vi "Periodic Tasks.vi"(8 "error in":errorcluster) -> ()   [LabVIEW 2015]
doc: "This VI runs in parallel to other tasks. It can contain as many user-defined periodic loops as you need. These can carry out PID or other sorts of timed response."
uses:
  Common Code/Change Detect Int.vi
  Robot Global Data.vi
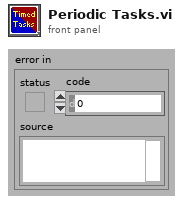
[diagram p1: front panel]
types:
  T1 = typedef "WPI_MotorControlDeviceRef.ctl" = cluster{"DeviceStatus":errorcluster, "Type":T2, "PWM":cluster{"PWM Channel":T3, "DeadBand":T4}, "CAN":cluster{"Device Number":u8, "Control Mode":T5, "Semaphore":T6, "Max Vout":dbl, "TalonSRX Control Mode":T7}, "Invert":bool}
  T2 = typedef "WPI_MotorControlType.ctl" = enum16{"PWM", "CAN", "CANTalonSRX"}
  T3 = typedef "FPGA_DIOPWMChannel.ctl" = enum8{"PWM 0", "PWM 1", "PWM 2", "PWM 3", "PWM 4", "PWM 5", "PWM 6", "PWM 7", "PWM 8", "PWM 9", "PWM MXP 0", "PWM MXP 1", "PWM MXP 2", "PWM MXP 3", "PWM MXP 4", "PWM MXP 5", "PWM MXP 6", "PWM MXP 7", "PWM MXP 8", "PWM MXP 9", "Invalid"}
  T4 = typedef "WPI_PWMDeadband.ctl" = cluster{"Name":string, "maxPositivePwm":i32, "minPositivePwm":i32, "centerPwm":i32, "maxNegativePwm":i32, "minNegativePwm":i32, "angularRange":u16}
  T5 = typedef "WPI_CANJaguar_ControlMode.ctl" = enum8{"Percent VBus", "Current", "Speed", "Position", "Voltage"}
  T6 = typedef "Semaphore RefNum" = refnum<k1>
  T7 = typedef "WPI_CANTalonSRX_APIControlMode.ctl" = enum8{"Percent VBus", "Speed", "Position", "Slave", "Unchanged / Invalid", "Voltage Compensation", "Current", "Motion Profile"}
  T8 = typedef "Dashboard Control Data.ctl" = cluster{"Shooter Presets":T9, "Encoder Control":T11, "Steer PID output":cluster{"output high":dbl, "output low":dbl}, " Steer PID gains":cluster{"proportional gain (Kc)":dbl, "integral time (Ti, min)":dbl, "derivative time (Td, min)":dbl}, "Drivetrain Settings":T12, "Vision Packet":T13, "Dashboard Drivetrain Command":T14, "Info/Command Cluster":T16, "Ball Vision Packet":T17, "Intake Presets":T19, "Intake Encoder Control":T21, "Climb Presets":T22, "Ultrasonic Limit":dbl, "Roll Limit":dbl, "Pitch Limit":dbl, "Goal Output Range":cluster{"output high":dbl, "output low":dbl}, "Enabled Systems":T23}
  T9 = typedef "Shooter Presets.ctl" = cluster{"Batter Shot":T10, "Deep Middle Shot":T10, "Manual Shot":T10, "Left Ticks Per Rotation":dbl, "Right Ticks Per Rotation":dbl, "Low Bar Shot":T10, "Shooter RPM Tolerance":dbl, "IIR Filter Power":dbl, "Trigger Power":dbl, "Fire from Load Delay":i32, "Max Angle":dbl, "Min Angle":dbl, "Angle PID gains":cluster{"P":dbl, "I":dbl, "D":dbl}, "Angle Output":cluster{"output high":dbl, "output low":dbl}, "Shooter Angle Tolerance":dbl, "Vision Shoot x^2":dbl, "Vision Shoot x":dbl, "Dist from Axis Cam to Pivot":dbl, "High Goal Center Height":dbl, "Feed Forward Max Accel":dbl, "Feed Forward Kv":dbl, "Backwards Trigger":dbl, "Shot Finish Delay (ms)":dbl, "Angle Max Current":dbl, "Angle Current Trip Time":dbl, "Intake Angle":dbl, "Vision Shoot c":dbl, "Reset?":bool, "Servo Release Delay":dbl, "Servo Idle Angle":i32, "Servo Hold Angle":i32, "Angle Pot x":dbl, "Angle Pot c":dbl, "Ignore Angle?":bool, "Manual Output?":bool, "Manual Out":dbl, "Max RPM":dbl, "Safty Frist Angle":dbl, "Intake Danger Height":dbl, "Angle Pot B":i32, "Angle Pot M":dbl, "FF Finish RPM":dbl, "RPM PID Right":cluster{"P":dbl, "I":dbl, "D":dbl, "FF":dbl}, "RPM PID Left":cluster{"P":dbl, "I":dbl, "D":dbl, "FF":dbl}}
  T10 = typedef "Shot Presets.ctl" = cluster{"Left":dbl, "Right":dbl, "Angle":dbl}
  T11 = typedef "Encoder Control.ctl" = cluster{"Right Tick Constant":dbl, "Left Tick Constant":dbl, "Reset?":bool, "Y Dist":cluster{"PID gains":cluster{"proportional gain (Kc)":dbl, "integral time (Ti, min)":dbl, "derivative time (Td, min)":dbl}}, "Y Stop Thresh":dbl, "Y Stop Speed":dbl}
  T12 = typedef "Drivetrain Settings.ctl" = cluster{"Gyro Tolerance":dbl, "Throttle Ramp (ms)":dbl, "Angular rate compensation":bool, "Throttle to Rate Scale":dbl, "Rate compensation gain":dbl, "Kv":dbl, "Ka":dbl, "Feed Forward P":dbl, "Feed Forward D":dbl, "Goal Vision PID gains":cluster{"proportional gain (Kc)":dbl, "integral time (Ti, min)":dbl, "derivative time (Td, min)":dbl}, "Goal Detection Window":dbl}
  T13 = typedef "Goal Vision Packet.ctl" = cluster{"Distance":dbl, "Center X":dbl, "Center Y":dbl, "Found Target?":bool}
  T14 = typedef "Dashboard Drivetrain Command.ctl" = cluster{"Drivetrain Vision":T15}
  T15 = typedef "Drivetrain Vision.ctl" = cluster{"Goal Window":dbl, "Ball Window":dbl}
  T16 = typedef "Ball Tracking Command Cluster.ctl" = cluster{"Distance to Ball":dbl, "Desired Angle":dbl, "Command":enum16{"Turn to Ball", "Turn to Angle", "Get Distance"}, "Pixels from Center":dbl}
  T17 = typedef "Ball Vision Packet.ctl" = cluster{"Ball Detected?":bool, "Distance to Ball":dbl, "Desired Angle":dbl, "Pixels from Center":dbl, "Tracking mode":T18}
  T18 = typedef "Tracking Mode.ctl" = enum16{"Turn to Ball", "Turn to Angle"}
  T19 = typedef "Intake Presets.ctl" = cluster{"Intake Speed":dbl, "Outake Speed":dbl, "Low Height":dbl, "Half Height":dbl, "Full Height":dbl, "Angle Speed":dbl, "Angle Tolerance":dbl, "Encoder Scale":dbl, "Load Height":dbl, "Output Range":T20, "Rotation Power Max/Min":dbl, "MaxCurrent":dbl, "Intake Trip Time":dbl, "Idle Height":dbl, "Max Height":dbl, "Reset Encoders?":bool, "PID gains":cluster{"proportional gain (Kc)":dbl, "integral time (Ti, min)":dbl, "derivative time (Td, min)":dbl}}
  T20 = typedef "Drivetrain Output Range.ctl" = cluster{"output high":dbl, "output low":dbl}
  T21 = typedef "IntakeEcoderControl.ctl" = cluster{"Arm Tick Constant":dbl, "Reset?":bool, "Y Dist":cluster{"PID gains":cluster{"proportional gain (Kc)":dbl, "integral time (Ti, min)":dbl, "derivative time (Td, min)":dbl}}, "Y Stop Thresh":dbl, "Y Stop Speed":dbl}
  T22 = typedef "Climb Presets.ctl" = cluster{"Pull Power":dbl, "Unpin Power":dbl, "Time to Hold":dbl}
  T23 = typedef "Enabled Systems.ctl" = cluster{"Shoot":bool, "Intake":bool, "DT":bool, "Gyro":bool, "100ms":bool, "US":bool}
  T24 = typedef "WPI_DriverStationRobotMode2.ctl" = enum16{"Autonomous Disabled", "Autonomous Enabled", "Teleop Disabled", "Teleop Enabled", "Disconnected", "Finish", "Test Disabled", "Test Enabled", "Emergency Stopped"}
  T25 = typedef "Shooter State Cluster.ctl" = cluster{"State":T26, "Left RPM":dbl, "Right RPM":dbl, "Shooter Ready?":bool, "Ball Loaded?":bool, "Current Angle":dbl, "Angle Motor Output":dbl, "Trigger Output":dbl, "Angle Ready?":bool, "RPM Ready?":bool, "Vision Ready?":bool, "Ball Loaded?":bool, "Mode":T27, "Shot Type":T28, "Pot Height":dbl, "Current Tripped Forward?":bool, "Current Tripped Backward?":bool, "Right Servo":i32, "Left Servo":i32}
  T26 = typedef "Shooter State.ctl" = enum16{"Idle", "Warmup", "Shooter Ready", "Shoot"}
  T27 = typedef "Shoot Modes Enum.ctl" = enum16{"Manual", "Safe", "Auto"}
  T28 = typedef "Shot Type.ctl" = enum16{"Batter Shot", "Corner Shot", "Curve Shot", "Vision Shot", "Deep Middle Shot"}
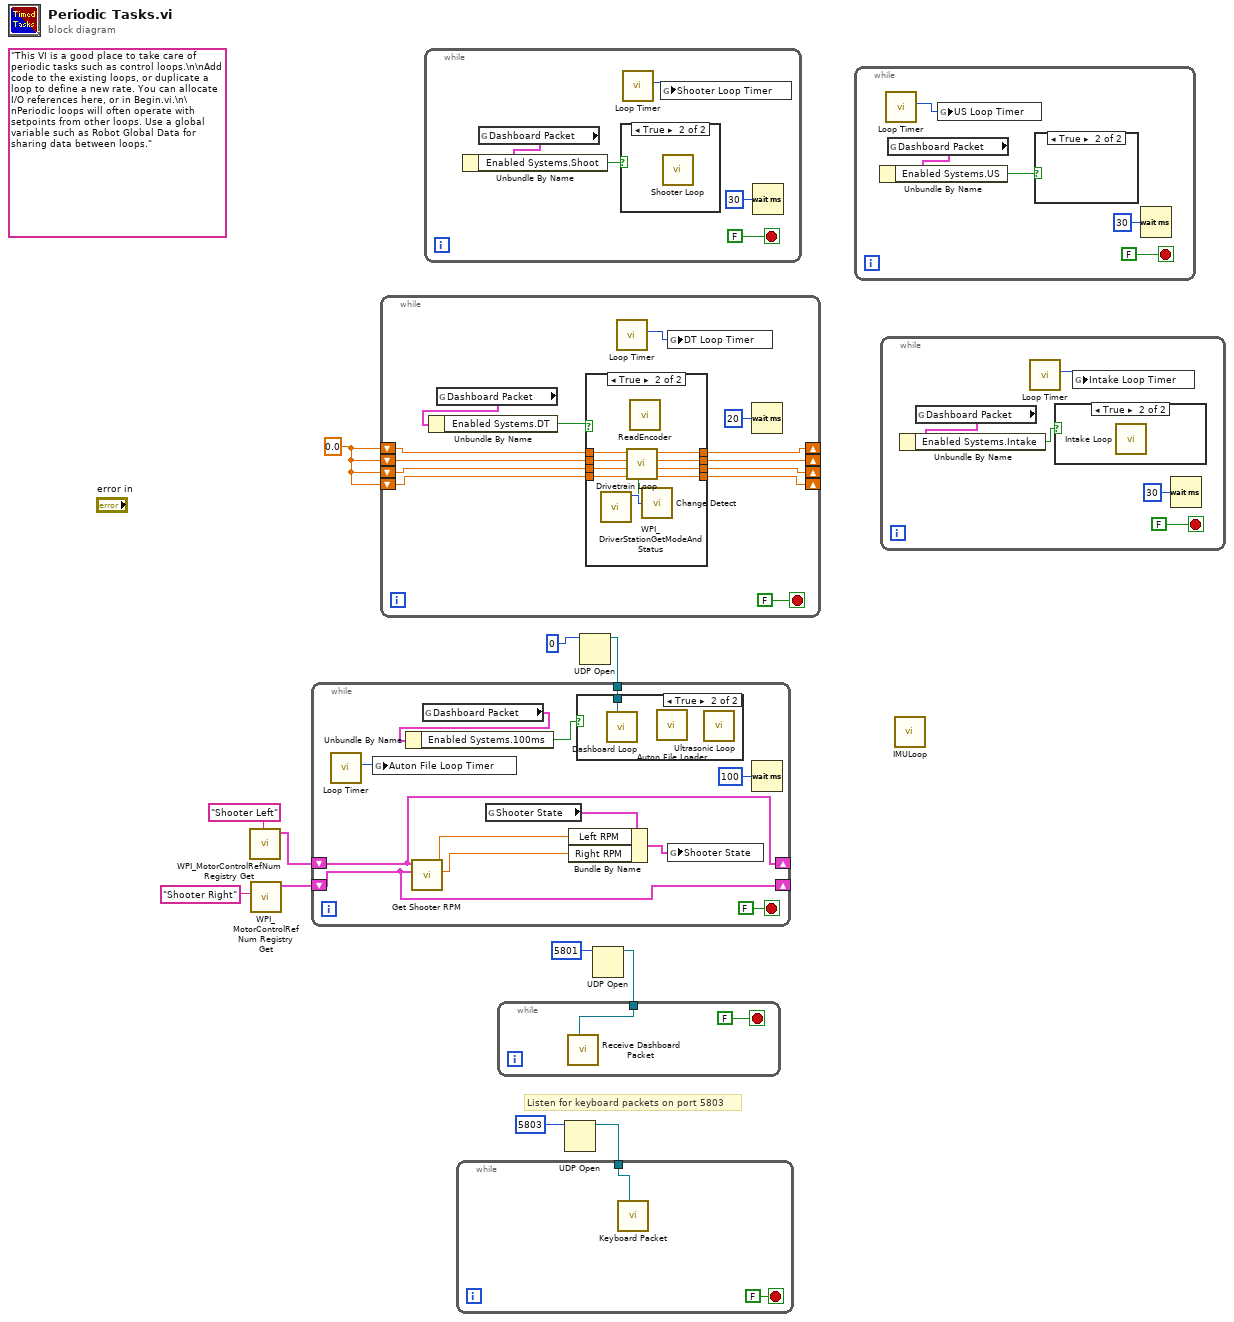
[diagram p0: block diagram]
diagram:
  w5 = 0.0 ("Timer 1 out")
  (unwired) "This VI is a good place to take care of periodic tasks such as control loops.\n\nAdd code to the existing loops, or duplicate a loop to define a new rate. You can allocate I/O references here, or in Begin.vi.\n\nPeriodic loops will often operate with setpoints from other loops. Use a global variable such as Robot Global Data for sharing data between loops."
  # "Listen for keyboard packets on port 5803"
  n1 = call <vilib>:"WPI_MotorControlRefNum Registry Get.vi"("refnum name"="Shooter Left") -> ("MotorControlDevRef"=w1:T1)  [unwired: 9 in, 1 out]
  n2 = call <vilib>:"WPI_MotorControlRefNum Registry Get.vi"("refnum name"="Shooter Right") -> ("MotorControlDevRef"=w2:T1)  [unwired: 9 in, 1 out]
  n3 = while {
    shift-right: [w17] -> _
    shift-left: w5 -> [w18]
    shift-right: [w21] -> _
    shift-left: w5 -> [w22]
    shift-right: [w16] -> _
    shift-left: w5 -> [w20]
    shift-right: [w15] -> _
    shift-left: w5 -> [w19]
    stop <- FALSE stop-if-true
    n4 = global read "Robot Global Data.vi" "Dashboard Packet"() -> (w13:T8)
    n5 = Unbundle By Name(w13) -> ("Enabled Systems.DT"=w12:bool)
    n6 = case shown="True" w12 {
      tunnel: w22 -> [w27 w37]
      tunnel: [w27 w36] -> w21
      tunnel: w20 -> [w26 w35]
      tunnel: w19 -> [w25 w34]
      tunnel: w18 -> [w28 w33]
      tunnel: [w28 w32] -> w17
      tunnel: [w26 w31] -> w16
      tunnel: [w25 w30] -> w15
      frame False {
      }
      frame True {
        n7 = call <vilib>:"WPI_DriverStationGetModeAndStatus.vi"() -> ("Robot Mode"=w38:T24)  [unwired: 10 in, 1 out]
        n8 = call "ReadEncoder.vi"() -> ()  [unwired: 11 in, 1 out]
        n9 = call-poly "Change Detect.vi"("In"=w38) -> ("Changed?"=w29:bool)
        n10 = call "Drivetrain Loop.vi"("Reset the clock"=w29, "In 4"=w34, "In 3"=w35, "In 2"=w37, "In 1"=w33) -> ("Out 4"=w30:dbl, "Out 3"=w31:dbl, "Out 2"=w36:dbl, "Out 1"=w32:dbl)  [unwired: 3 in]
      }
    }
    n11 = call "Loop Timer.vi"() -> ("dt"=w14:u32)  [unwired: 11 in]
    n12 = global write "Robot Global Data.vi" "DT Loop Timer"(w14) -> ()
    n13 = Wait (ms)(milliseconds to wait=u32 20) -> ()  [unwired: 1 out]
  }
  n14 = while {
    stop <- FALSE stop-if-true
    n15 = global read "Robot Global Data.vi" "Dashboard Packet"() -> (w40:T8)
    n16 = Unbundle By Name(w40) -> ("Enabled Systems.Shoot"=w39:bool)
    n17 = case shown="True" w39 {
      frame False {
      }
      frame True {
        n18 = call "Shooter Loop.vi"() -> ()  [unwired: 12 in]
      }
    }
    n19 = call "Loop Timer.vi"() -> ("dt"=w41:u32)  [unwired: 11 in]
    n20 = global write "Robot Global Data.vi" "Shooter Loop Timer"(w41) -> ()
    n21 = Wait (ms)(milliseconds to wait=u32 30) -> ()  [unwired: 1 out]
  }
  n22 = UDP Open(11:u16 5803 ("port")) -> (port=w6:refnum<k16>)  [unwired: 4 in, 2 out]
  n23 = while {
    tunnel: w6 -> [w44]
    stop <- FALSE stop-if-true
    n24 = call "Keyboard Packet.vi"("connection ID"=w44) -> ()  [unwired: 11 in]
  }
  n25 = UDP Open(11:0) -> (port=w9:refnum<k16>)  [unwired: 4 in, 2 out]
  n26 = while {
    tunnel: w9 -> [w55]
    shift-right: [w46] -> _
    shift-left: w1 -> [w46]
    shift-right: [w47] -> _
    shift-left: w2 -> [w47]
    stop <- FALSE stop-if-true
    n27 = call "Loop Timer.vi"() -> ("dt"=w54:u32)  [unwired: 11 in]
    n28 = global write "Robot Global Data.vi" "Auton File Loop Timer"(w54) -> ()
    n29 = call "Get Shooter RPM.vi"("Shooter Right"=w47, "Shooter Left"=w46) -> ("Right RPM"=w49:dbl, "Left RPM"=w50:dbl)  [unwired: 5 in, 3 out]
    n30 = global read "Robot Global Data.vi" "Dashboard Packet"() -> (w53:T8)
    n31 = Unbundle By Name(w53) -> ("Enabled Systems.100ms"=w52:bool)
    n32 = global read "Robot Global Data.vi" "Shooter State"() -> (w51:T25)
    n33 = Bundle By Name(cluster=w51, "Left RPM"=w50, "Right RPM"=w49) -> (w48:T25)
    n34 = case shown="True" w52 {
      tunnel: w55 -> [_ w58]
      frame False {
      }
      frame True {
        n35 = call "Dashboard Loop.VI"("connection ID"=w58) -> ()  [unwired: 11 in]
        n36 = call "Auton File Loader.vi"() -> ()  [unwired: 12 in]
        n37 = call "Ultrasonic Loop.vi"() -> ()  [unwired: 12 in]
      }
    }
    n38 = global write "Robot Global Data.vi" "Shooter State"(w48) -> ()
    n39 = Wait (ms)(milliseconds to wait=u32 100) -> ()  [unwired: 1 out]
  }
  n40 = UDP Open(11:u16 5801 ("port")) -> (port=w11:refnum<k16>)  [unwired: 4 in, 2 out]
  n41 = while {
    tunnel: w11 -> [w59]
    stop <- FALSE stop-if-true
    n42 = call "Receive Dashboard Packet.vi"("connection ID"=w59) -> ()  [unwired: 11 in]
  }
  n43 = while {
    stop <- FALSE stop-if-true
    n44 = call "Loop Timer.vi"() -> ("dt"=w63:u32)  [unwired: 11 in]
    n45 = global read "Robot Global Data.vi" "Dashboard Packet"() -> (w62:T8)
    n46 = Unbundle By Name(w62) -> ("Enabled Systems.US"=w61:bool)
    n47 = global write "Robot Global Data.vi" "US Loop Timer"(w63) -> ()
    n48 = case shown="True" w61 {
      frame False {
      }
      frame True {
      }
    }
    n49 = Wait (ms)(milliseconds to wait=u32 30) -> ()  [unwired: 1 out]
  }
  n50 = while {
    stop <- FALSE stop-if-true
    n51 = global read "Robot Global Data.vi" "Dashboard Packet"() -> (w67:T8)
    n52 = Unbundle By Name(w67) -> ("Enabled Systems.Intake"=w66:bool)
    n53 = call "Loop Timer.vi"() -> ("dt"=w68:u32)  [unwired: 11 in]
    n54 = case shown="True" w66 {
      frame False {
      }
      frame True {
        n55 = call "Intake Loop.vi"() -> ()  [unwired: 12 in]
      }
    }
    n56 = global write "Robot Global Data.vi" "Intake Loop Timer"(w68) -> ()
    n57 = Wait (ms)(milliseconds to wait=u32 30) -> ()  [unwired: 1 out]
  }
  n58 = call "IMULoop.vi"() -> ()  [unwired: 12 in]
